vi "read ave pH July 2016 v1_0.vi"() -> (0 "Ave pH":dbl caption="Scaled Single Value" format="%#.1g")   [LabVIEW 2012]
uses:
  Instance           1 19Saved   read ave pH .vi
  Instance           4 19Saved   read ave pH .vi
  <vilib>/measure/madcrms.llb/Averaged DC-RMS for 1 Chan.vi
  <vilib>/measure/NI_MAPro.lvlib
panel:
  out "Waveform Chart":dbl(graph)
  in  "Y-Intercept":dbl=13.8
  in  "Slope":dbl=-3.85
  in  "Offset":dbl min=-1.0 max=1.0 step=0.01
  out "RMS Ave Volt":dbl[](array[numeric])=[2.5340775185610775] format="%#.3g"
  out "Ave Volt":dbl[](array[numeric])=[2.53407748191501] format="%#.3g"
  in  "Channel":i32
  # "N- points measurement -- intended to be used as a subVI\nbut left outside the suvVI folder to double as a simple pH check\n- \"printing\" also the raw signal for diagnostic\n- Terminal set to have one connection -- the average value\n- The sensor is hardwired to pH in the wiring diagram\n\nDerived from \"read pH\" -- now averaging a wave in case the\ninput is noisy"
  # "When you use it as a simple diagnostic tool, use the run continuously mode"
  # "Calibration Inputs"
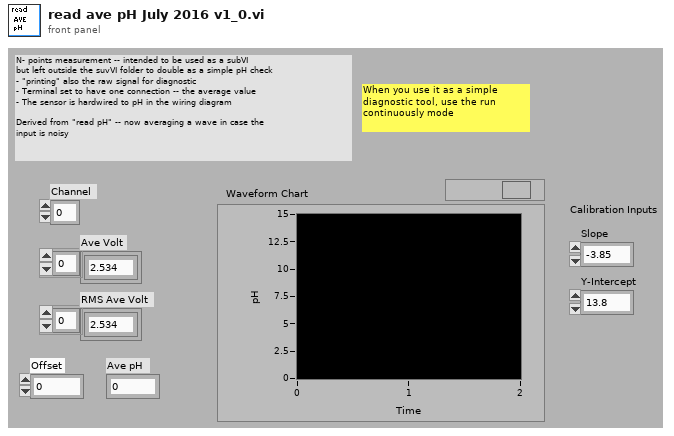
[diagram p1: front panel]
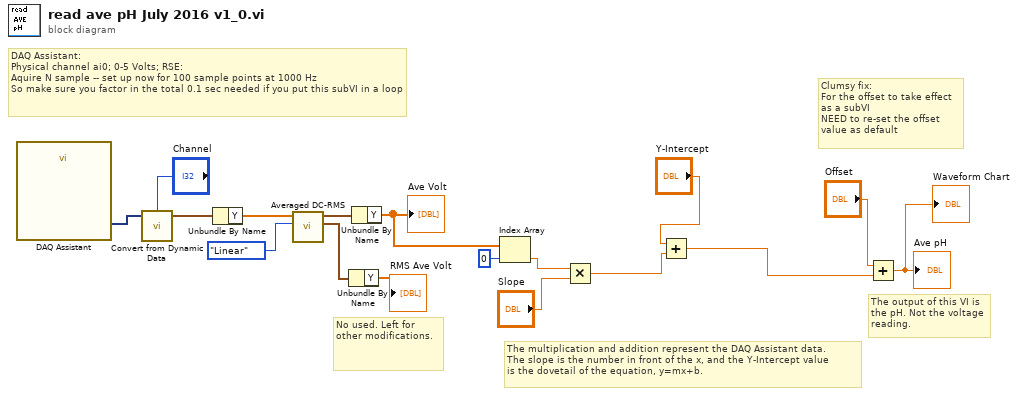
[diagram p0: block diagram]
diagram:
  # "The multiplication and addition represent the DAQ Assistant data.\nThe slope is the number in front of the x, and the Y-Intercept value \nis the dovetail of the equation, y=mx+b."
  # "Clumsy fix:\nFor the offset to take effect as a subVI\nNEED to re-set the offset value as default"
  # "The output of this VI is the pH. Not the voltage reading."
  # "No used. Left for other modifications."
  # "DAQ Assistant: \nPhysical channel ai0; 0-5 Volts; RSE: \nAquire N sample -- set up now for 100 sample points at 1000 Hz\nSo make sure you factor in the total 0.1 sec needed if you put this subVI in a loop"
  n1 = call "DAQ Assistant"() -> ("data"=w17:dynamicdata)  [unwired: 17 in, 2 out]
  n2 = call "Convert from Dynamic Data"("Dynamic Data Type"=w17, "Channel"="Channel") -> ("Waveform"=w16:waveform(dbl))  [unwired: 2 in]
  n3 = Unbundle By Name(w16) -> ("Y"=w14:dbl[])
  n4 = call-poly <vilib>:"Averaged DC-RMS.vi"("averaging type"=enum16{"Linear", "Exponential"}."Linear", "signal in"=w14) -> ("RMS value waveform"=w11:waveform(dbl), "DC value waveform"=w12:waveform(dbl))  [unwired: 5 in, 3 out]
  n5 = Unbundle By Name(w11) -> ("Y"=→"RMS Ave Volt":dbl[])
  n6 = Unbundle By Name(w12) -> ("Y"=w2:dbl[])
  "Ave Volt" <- w2
  n7 = Index Array(array=w2, index=0) -> (element=w7:dbl)
  n8 = Multiply(x=w7, y="Slope") -> (x*y=w5:dbl)
  n9 = Add(x="Y-Intercept", y=w5) -> (x+y=w3:dbl)
  n10 = Add(x="Offset", y=w3) -> (x+y=→"Ave pH" →"Waveform Chart":dbl)
